vi "toCluster.vi"(8 "error in (no error)":errorcluster, 11 "ACNET Device in":refnum<class "ACNET Device.lvclass">) -> (0 "error out":errorcluster, 2 "ACNET Device Cluster":T1, 3 "ACNET Device out":refnum<class "ACNET Device.lvclass">)   [LabVIEW 2013, in "ACNET Monitor.lvlib" / "ACNET Device.lvclass"]
uses:
  ACNET Device.lvclass
  ACNET Device.lvclass/ACNET Device.ctl
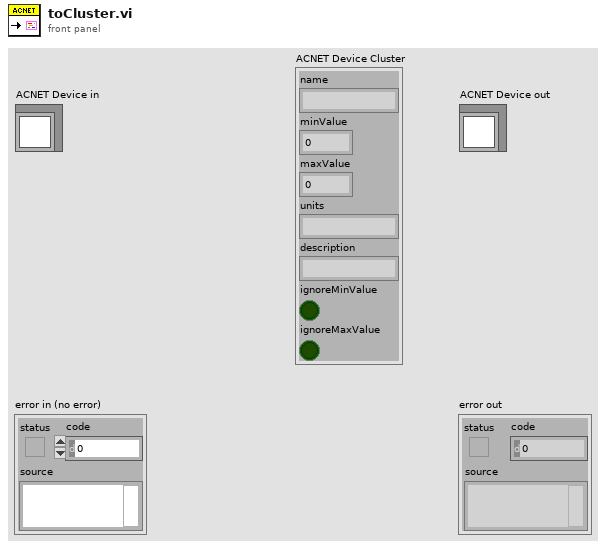
[diagram p1: front panel]
types:
  T1 = cluster{"name":string, "minValue":dbl, "maxValue":dbl, "units":string, "description":string, "ignoreMinValue":bool, "ignoreMaxValue":bool}
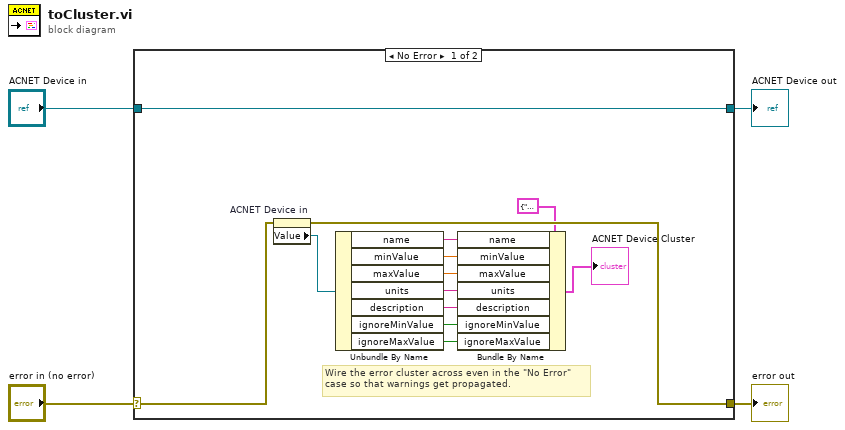
[diagram p0: block diagram]
diagram:
  n1 = case shown="No Error" "error in (no error)" {
    selector: "error in (no error)" -> [w16 w19]
    tunnel: [w15 w19] -> w3
    tunnel: [w17 w18] -> w1
    tunnel: "ACNET Device in" -> [w17 w18]
    frame No Error {
      # "Wire the error cluster across even in the \"No Error\"\ncase so that warnings get propagated."
      n2 = property on="ACNET Device in" class="LVClassControl (strict)"(error in=w16) -> (error out=w15:errorcluster, "Value"=w11:refnum<class "ACNET Device.lvclass">)  [unwired: 1 in, 1 out]
      n3 = Unbundle By Name(w11) -> ("name"=w14:string, "minValue"=w13:dbl, "maxValue"=w12:dbl, "units"=w10:string, "description"=w7:string, "ignoreMinValue"=w6:bool, "ignoreMaxValue"=w5:bool)
      n4 = Bundle By Name(cluster=T1 {"name"="", "minValue"=0.0, "maxValue"=0.0, "units"="", "description"="", "ignoreMinValue"=FALSE, "ignoreMaxValue"=FALSE} ("ACNET Device Cluster"), "name"=w14, "minValue"=w13, "maxValue"=w12, "units"=w10, "description"=w7, "ignoreMinValue"=w6, "ignoreMaxValue"=w5) -> (→"ACNET Device Cluster":T1)
    }
    frame Error {
    }
  }
  "error out" <- w3
  "ACNET Device out" <- w1
